vi "Constants.vi"() -> ()   [LabVIEW 2014, in "NIAnalysis.lvlib"]
uses:
  NIAnalysis.lvlib
panel:
  in  "App.Sufix":string=".AppVersion"
  in  "Boot.Sufix":string=".BootVersion"
  in  "LT.AnalyzeChannel":string="LT.AnalyzeChannel"
  in  "LIN2.Sufix":string=".LIN2.Result"
  in  "LIN1.Sufix":string=".LIN1.Result"
  in  "VBATT.Property":string="VBATTLevel"
  in  "Fault.Sufix":string=".Fault.Result"
  in  "FaultReq.Sufix":string="_Fault_Type_Req"
  in  "FaultType.Sufix":string="_Fault_Type"
  in  "Fault.Folder":string="Fault Status"
  in  "SN.Sufix":string=".SerialNumber"
  in  "LT.Sufix":string=".LevelTransition.Result"
  in  "VS Group":string="VeriStand Channels"
  in  "Rate.Property":string="LogRate"
  in  "DMM.Sufix":string=".SleepMeasurement.Result"
  in  "Iteration.Property":string="Iteration"
  in  "CSV.Property":string="CSVStimulus.Path"
  in  "Cycled.Sufix":string=".Cycled"
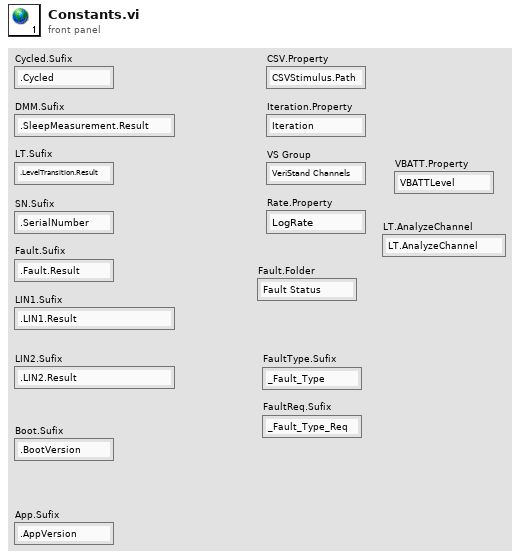
[diagram p1: front panel]
diagram:
